vi "MonitoringDemo.vi"() -> ()   [LabVIEW 2020]
panel:
  in  "Command":string
  in  "Send_command":bool
  in  "Send Stop":bool
  out "gamma":dbl
  out "beta":dbl
  out "alpha":dbl
  out "z":dbl
  out "y":dbl
  out "x":dbl
  out "J6":dbl
  out "J5":dbl
  out "J4":dbl
  out "J3":dbl
  out "J2":dbl
  out "J1":dbl
  in  "stop":bool
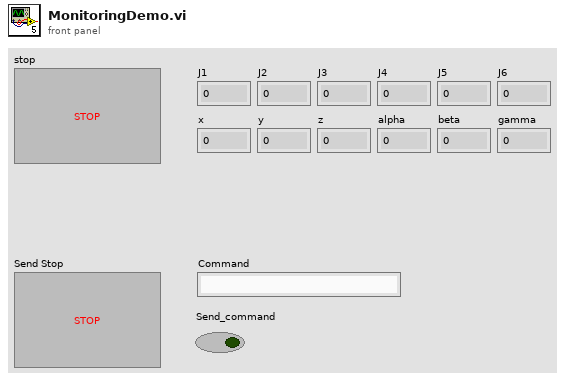
[diagram p1: front panel]
types:
  T1 = enum16{"Standard", "Buffered", "CRLF", "Immediate"}
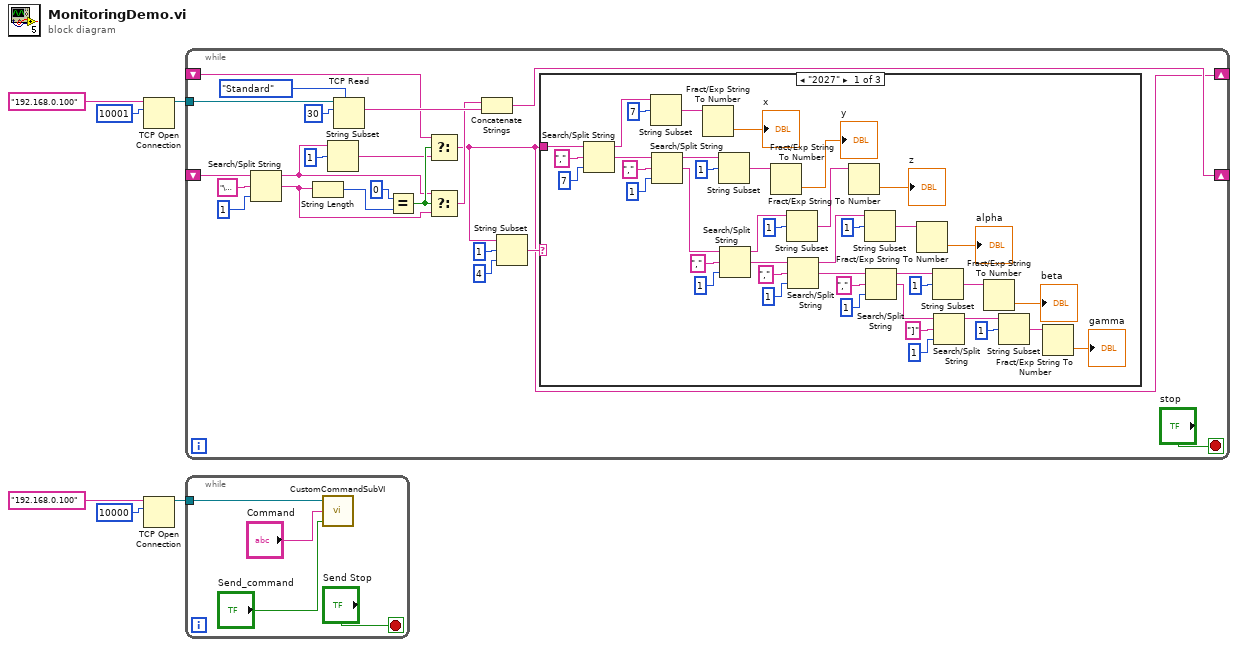
[diagram p0: block diagram]
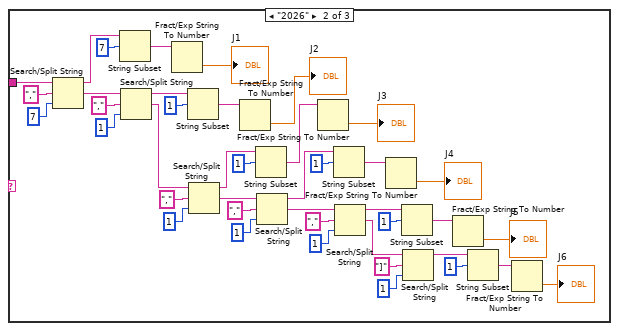
[diagram p2: hidden frame]
diagram:
  n1 = TCP Open Connection(address="192.168.0.100", remote port or service name=u16 10001) -> (connection ID=w4:refnum<k5>)  [unwired: 3 in, 1 out]
  n2 = TCP Open Connection(address="192.168.0.100", remote port or service name=u16 10000) -> (connection ID=w1:refnum<k5>)  [unwired: 3 in, 1 out]
  n3 = while {
    tunnel: w4 -> [w28]
    shift-right: [w21] -> _
    shift-left: _ -> [w22]
    shift-right: [w7] -> _
    shift-left: _ -> [w8]
    stop <- "stop" stop-if-true
    n4 = Search/Split String(string=w22, search string/char (-)="\u0000", offset (0)=1) -> (substring before match=w13:string, match + rest of string=w15:string)  [unwired: 1 out]
    n5 = String Length(string=w15) -> (length=w18:i32)
    n6 = String Subset(string=w13, offset (0)=1) -> (substring=w12:string)  [unwired: 1 in]
    n7 = TCP Read(connection ID=w28, bytes to read=30, 7:T1."Standard" ("mode (standard)")) -> (data out=w24:string)  [unwired: 2 in, 2 out]
    n8 = Equal?(x=0, y=w18) -> (x = y?=w14:bool)
    n9 = Select(t=w8, s=w14, f=w12) -> (s? t:f=w7:string)
    n10 = Select(t=w13, s=w14, f=w15) -> (s? t:f=w16:string)
    n11 = Concatenate Strings(w16, w24) -> (w21:string)
    n12 = String Subset(string=w7, offset (0)=1, length (rest)=4 ("length (rest)")) -> (substring=w9:string)
    n13 = case shown="\"2027\"" w9 {
      tunnel: w7 -> [w29 w112 _]
      frame "2027" {
        n14 = Search/Split String(string=w29, search string/char (-)=",", offset (0)=7) -> (substring before match=w68:string, match + rest of string=w66:string)  [unwired: 1 out]
        n15 = String Subset(string=w68, offset (0)=7) -> (substring=w35:string)  [unwired: 1 in]
        n16 = Search/Split String(string=w66, search string/char (-)=",", offset (0)=1) -> (substring before match=w52:string, match + rest of string=w61:string)  [unwired: 1 out]
        n17 = Fract/Exp String To Number(string=w35) -> (number=→"x":dbl)  [unwired: 3 in, 1 out]
        n18 = String Subset(string=w52, offset (0)=1) -> (substring=w34:string)  [unwired: 1 in]
        n19 = Search/Split String(string=w61, search string/char (-)=",", offset (0)=1) -> (substring before match=w51:string, match + rest of string=w54:string)  [unwired: 1 out]
        n20 = Fract/Exp String To Number(string=w34) -> (number=→"y":dbl)  [unwired: 3 in, 1 out]
        n21 = String Subset(string=w51, offset (0)=1) -> (substring=w33:string)  [unwired: 1 in]
        n22 = Search/Split String(string=w54, search string/char (-)=",", offset (0)=1) -> (substring before match=w50:string, match + rest of string=w53:string)  [unwired: 1 out]
        n23 = Fract/Exp String To Number(string=w33) -> (number=→"z":dbl)  [unwired: 3 in, 1 out]
        n24 = String Subset(string=w50, offset (0)=1) -> (substring=w32:string)  [unwired: 1 in]
        n25 = Search/Split String(string=w53, search string/char (-)=",", offset (0)=1) -> (substring before match=w49:string, match + rest of string=w47:string)  [unwired: 1 out]
        n26 = Fract/Exp String To Number(string=w32) -> (number=→"alpha":dbl)  [unwired: 3 in, 1 out]
        n27 = String Subset(string=w49, offset (0)=1) -> (substring=w31:string)  [unwired: 1 in]
        n28 = Search/Split String(string=w47, search string/char (-)="]", offset (0)=1) -> (substring before match=w48:string)  [unwired: 2 out]
        n29 = Fract/Exp String To Number(string=w31) -> (number=→"beta":dbl)  [unwired: 3 in, 1 out]
        n30 = String Subset(string=w48, offset (0)=1) -> (substring=w30:string)  [unwired: 1 in]
        n31 = Fract/Exp String To Number(string=w30) -> (number=→"gamma":dbl)  [unwired: 3 in, 1 out]
      }
      frame "2026" {
        n32 = Search/Split String(string=w112, search string/char (-)=",", offset (0)=7) -> (substring before match=w109:string, match + rest of string=w107:string)  [unwired: 1 out]
        n33 = String Subset(string=w109, offset (0)=7) -> (substring=w76:string)  [unwired: 1 in]
        n34 = Search/Split String(string=w107, search string/char (-)=",", offset (0)=1) -> (substring before match=w93:string, match + rest of string=w102:string)  [unwired: 1 out]
        n35 = Fract/Exp String To Number(string=w76) -> (number=→"J1":dbl)  [unwired: 3 in, 1 out]
        n36 = String Subset(string=w93, offset (0)=1) -> (substring=w75:string)  [unwired: 1 in]
        n37 = Search/Split String(string=w102, search string/char (-)=",", offset (0)=1) -> (substring before match=w92:string, match + rest of string=w95:string)  [unwired: 1 out]
        n38 = Fract/Exp String To Number(string=w75) -> (number=→"J2":dbl)  [unwired: 3 in, 1 out]
        n39 = String Subset(string=w92, offset (0)=1) -> (substring=w74:string)  [unwired: 1 in]
        n40 = Search/Split String(string=w95, search string/char (-)=",", offset (0)=1) -> (substring before match=w91:string, match + rest of string=w94:string)  [unwired: 1 out]
        n41 = Fract/Exp String To Number(string=w74) -> (number=→"J3":dbl)  [unwired: 3 in, 1 out]
        n42 = String Subset(string=w91, offset (0)=1) -> (substring=w73:string)  [unwired: 1 in]
        n43 = Search/Split String(string=w94, search string/char (-)=",", offset (0)=1) -> (substring before match=w90:string, match + rest of string=w88:string)  [unwired: 1 out]
        n44 = Fract/Exp String To Number(string=w73) -> (number=→"J4":dbl)  [unwired: 3 in, 1 out]
        n45 = String Subset(string=w90, offset (0)=1) -> (substring=w72:string)  [unwired: 1 in]
        n46 = Search/Split String(string=w88, search string/char (-)="]", offset (0)=1) -> (substring before match=w89:string)  [unwired: 2 out]
        n47 = Fract/Exp String To Number(string=w72) -> (number=→"J5":dbl)  [unwired: 3 in, 1 out]
        n48 = String Subset(string=w89, offset (0)=1) -> (substring=w71:string)  [unwired: 1 in]
        n49 = Fract/Exp String To Number(string=w71) -> (number=→"J6":dbl)  [unwired: 3 in, 1 out]
      }
      frame Default {
      }
    }
  }
  n50 = while {
    tunnel: w1 -> [w114]
    stop <- "Send Stop" stop-if-true
    n51 = call "CustomCommandSubVI.vi"("Send_command"="Send_command", "Command"="Command", "TCP Network Connection in"=w114) -> ()  [unwired: 3 out]
  }
